vi "Q - not nan -- integer.vi"(8 "default":i32, 10 "Numeric":i32) -> (0 "Boolean":bool=TRUE, 2 "out":i32)   [LabVIEW 2018]
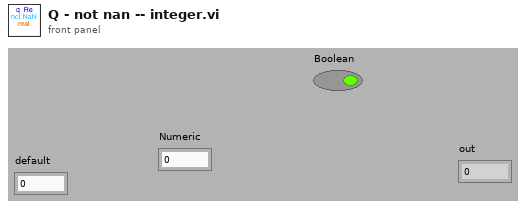
[diagram p1: front panel]
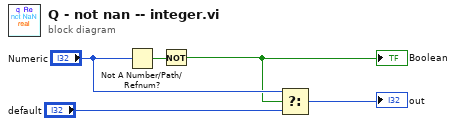
[diagram p0: block diagram]
diagram:
  n1 = Not A Number/Path/Refnum?(number/path/refnum="Numeric") -> (NaN/Path/Refnum?=w5:bool)
  n2 = Not(x=w5) -> (.not. x?=w1:bool)
  "Boolean" <- w1
  n3 = Select(t="Numeric", s=w1, f="default") -> (s? t:f=→"out":i32)
